vi "Open module.vi"(0 "Module":u16(ring)=5 items=["Atom removal 1", "Atom removal 2", "B-field off", "CMOT", "Defaults", "Final B-field ramps", "Fluorescence pulse", "High field", "High field ARP", "Loading cart QT", "Loading sci QT", "Low field", "Low field ARP", "Mol OD image", "Mol picture", "Mol probe pulse", "Molasses", "MOT off", "MOT on", "OD image", "Optical pumping", "OT B-field off", "Picture", "Probe pulse", "QT off for OT", "Quadrupole trap off", "Quadrupole trap", "Quantization axis", "S-G separation", "STIRAP back for imaging", "STIRAP", "TTL high", "TTL low", "GPIB", "Utility Module 1", "Utility Module 2", "Utility Module 3", "Utility Module 4", "Utility Module 5", "Utility Module 6", "Utility Module 7", "Utility Module 8", "Utility Module 9"]) -> ()   [LabVIEW 2017]
doc: "This vi opens the front panel of a selected module. It only works for modules with a specific connector pattern."
uses:
  globals/Modules global.vi
panel:
  in  "directory":string="C:\\Users\\BEC7\\Desktop\\New Experiment Control\\Modules\\"
  out "vi reference":refnum<vi>
  out "appended path":path=path "C:/Users/BEC7/Desktop/Project 1/Modules/Final B-field ramps.vi"
  in  "bottom":i16=600
  in  "right":i16=950
  in  "top":i16=81
  in  "left":i16=75
  in  "VI Type Specifier":refnum<vi>
  # "This subVI takes and input module (from a ring control) and opens the front panel."
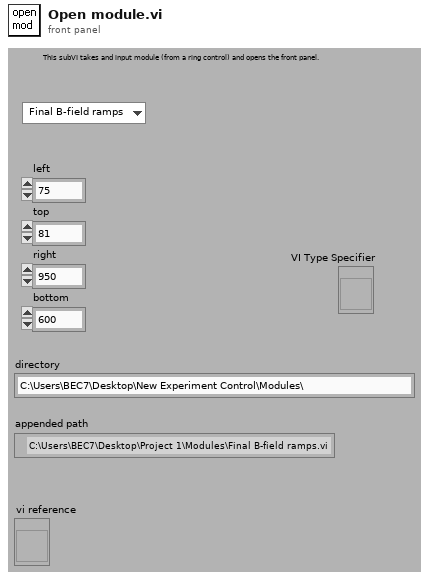
[diagram p1: front panel]
types:
  T1 = cluster{"left":i16, "top":i16, "right":i16, "bottom":i16}
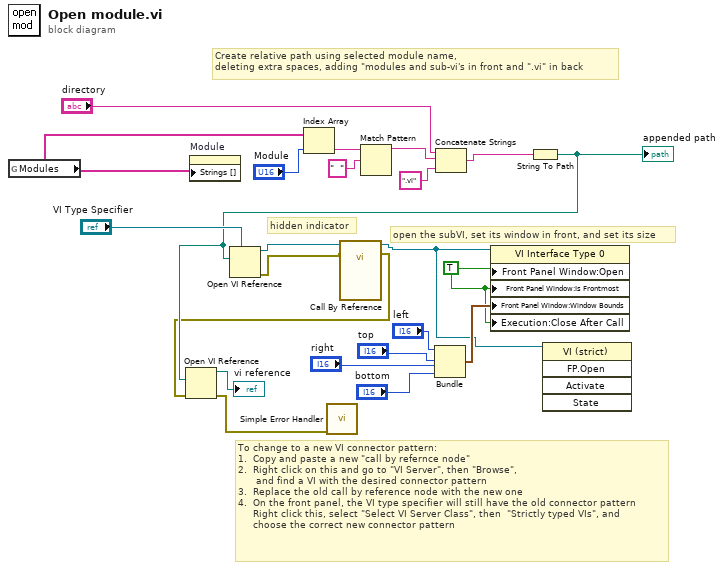
[diagram p0: block diagram]
diagram:
  w12 = TRUE ("Front Panel Window:Is Frontmost")
  # "To change to a new VI connector pattern: \n1.  Copy and paste a new \"call by refernce node\"\n2.  Right click on this and go to \"VI Server\", then \"Browse\",\n      and find a VI with the desired connector pattern\n3.  Replace the old call by reference node with the new one\n4.  On the front panel, the VI type specifier will still have the old connector pattern\n     Right click this, select \"Select VI Server Class\", then  \"Strictly typed VIs\", and\n     choose the correct new connector pattern"
  # "hidden indicator"
  # "open the subVI, set its window in front, and set its size"
  # "Create relative path using selected module name,\ndeleting extra spaces, adding \"modules and sub-vi's in front and \".vi\" in back"
  n1 = global read "Modules global.vi" "Modules"() -> (w17:string[])
  n2 = property on="Module" class="Ring (strict)"("Strings []"=w17) -> ()  [unwired: 2 in, 2 out]
  n3 = Index Array(array=w17, index="Module") -> (element=w14:string)
  n4 = Match Pattern(string=w14, regular expression="  ") -> (before substring=w13:string)  [unwired: 1 in, 3 out]
  n5 = Bundle("left"="left", "top"="top", "right"="right", "bottom"="bottom") -> (w21:T1)  [unwired: 1 in]
  n6 = Concatenate Strings("directory", w13, ".vi" ("string")) -> (w6:string)
  n7 = String To Path(string=w6) -> (path=w5:path)
  "appended path" <- w5
  n8 = Open VI Reference(type specifier VI Refnum (for type only)="VI Type Specifier", vi path=w5) -> (vi reference=w1:refnum<vi>, error out=w2:errorcluster)  [unwired: 4 in]
  n9 = call-by-ref "?"(reference=w1, error in=w2) -> (reference out=w4:refnum<vi>, error out=w3:errorcluster)  [unwired: 5 in, 3 out]
  n10 = Open VI Reference(vi path=w5, error in (no error)=w3) -> (vi reference=→"vi reference":refnum<vi>, error out=w7:errorcluster)  [unwired: 4 in]
  n11 = call <vilib>:"Simple Error Handler.vi"("error in (no error)"=w7) -> ()  [unwired: 4 in, 5 out]
  n12 = property class="VI Interface Type 0"(reference=w4, "Front Panel Window:Open"=w12, "Front Panel Window:Is Frontmost"=w12, "Front Panel Window:Window Bounds"=w21, "Execution:Close After Call"=w12) -> ()  [unwired: 1 in, 2 out]
  n13 = invoke class="VI (strict)" method="FP.Open"(reference=w4) -> ()  [unwired: 4 in, 5 out]
